vi "SetCurrentRange.vi"(8 "Error In":errorcluster, 9 "Expected Current (A)":dbl, 10 "Channel (1 or 2)":u8 min=1 max=2 step=1, 11 "Keithley 6482 In":refnum<visa-resource-name>) -> (0 "Error Out":errorcluster, 3 "Keithley 6482 Out":refnum<visa-resource-name>)   [LabVIEW 2009, in "Keithley-6482-Visa.lvlib"]
uses:
  <instrlib>/Keithley-6482-Visa9.0/Keithley-6482-Visa.lvlib
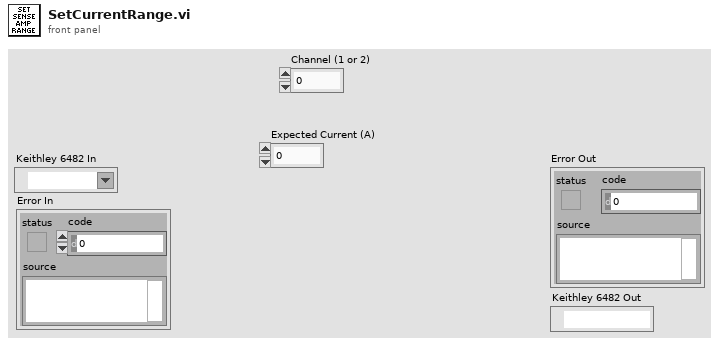
[diagram p1: front panel]
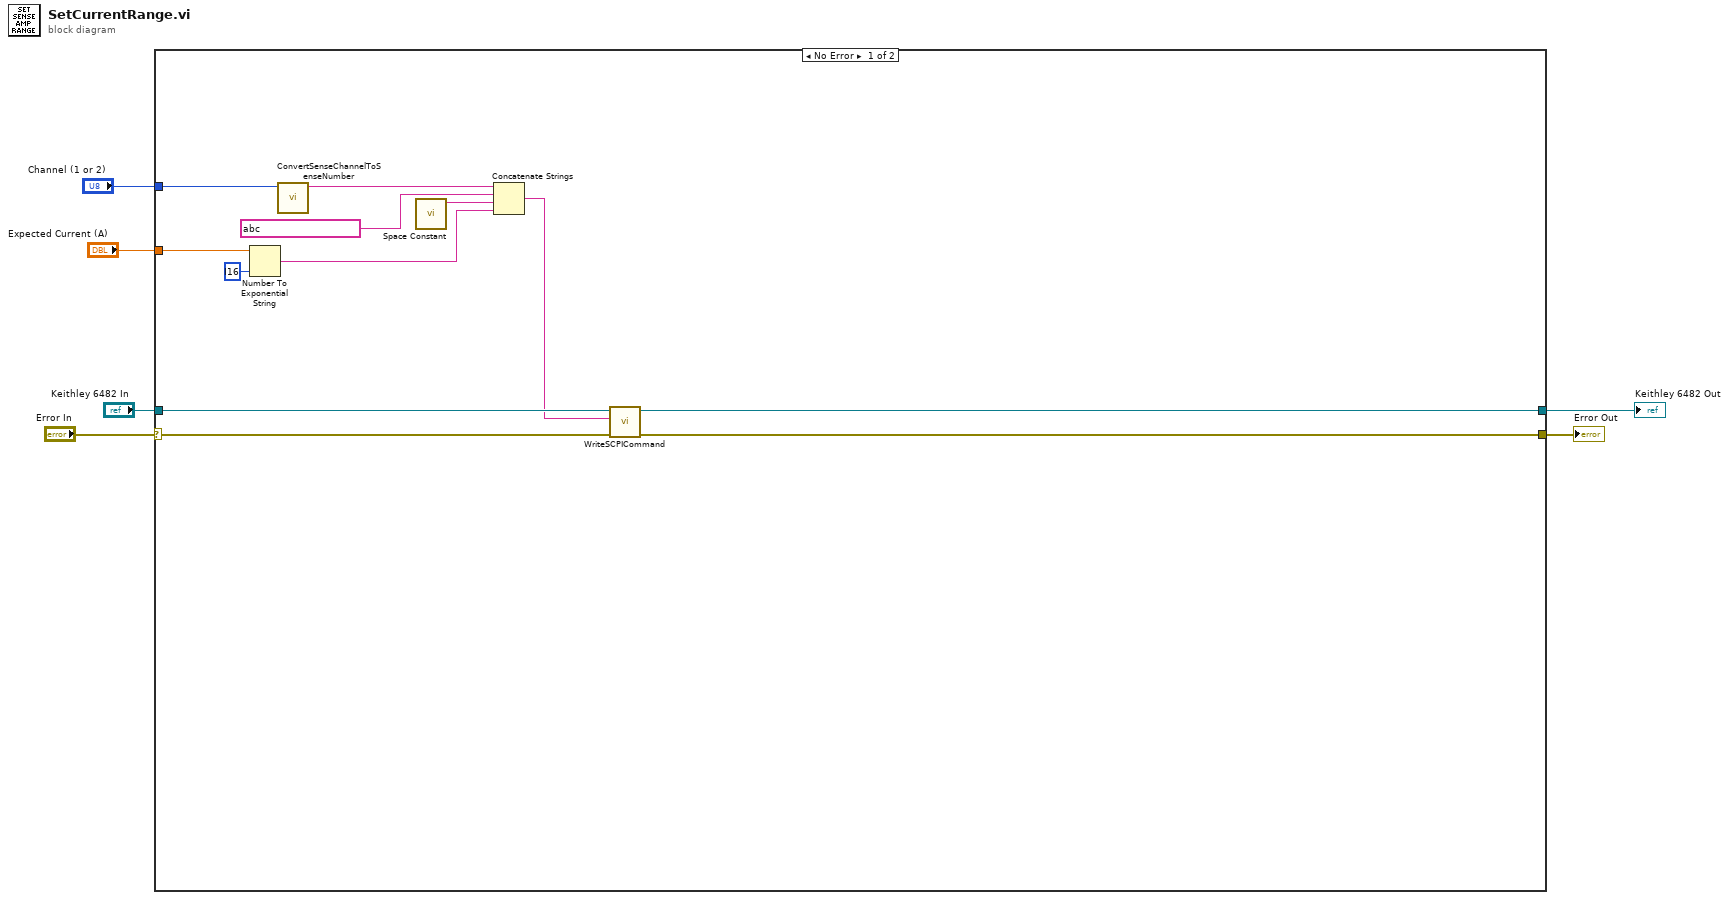
[diagram p0: block diagram]
diagram:
  n1 = case shown="No Error" "Error In" {
    selector: "Error In" -> [w18 w19]
    tunnel: "Keithley 6482 In" -> [w17 w20]
    tunnel: [w7 w19] -> w4
    tunnel: [w8 w20] -> w3
    tunnel: "Channel (1 or 2)" -> [w16 _]
    tunnel: "Expected Current (A)" -> [w12 _]
    frame #0 {
      n2 = Number To Exponential String(number=w12, precision (6)=i16 ?) -> (E-format string=w10:string)  [unwired: 2 in]
      n3 = call <instrlib>:"ConvertSenseChannelToSenseNumber.vi"("Channel (1 or 2)"=w16) -> ("Sense Number"=w15:string)  [unwired: 10 in]
      n4 = call <vilib>:"Space Constant.vi"() -> ("String"=w13:string)
      n5 = Concatenate Strings(w15, string ? ("string"), w13, w10) -> (w9:string)
      n6 = call <instrlib>:"WriteSCPICommand.vi"("Error In"=w18, "SCPI Command"=w9, "Keithley 6482 In"=w17) -> ("Error Out"=w7:errorcluster, "Keithley 6482 Out"=w8:refnum<visa-resource-name>)  [unwired: 7 in]
    }
    frame #1 {
    }
  }
  "Error Out" <- w4
  "Keithley 6482 Out" <- w3
